vi "Write Project Item.vi"(10 "Project Item":refnum<vi>, 11 "Target Store in":refnum<class "Target Store.lvclass">) -> (3 "Target Store out":refnum<class "Target Store.lvclass">)   [LabVIEW 2020, in "Add Actor.lvlib" / "Target Store.lvclass"]
uses:
  Target Store.lvclass
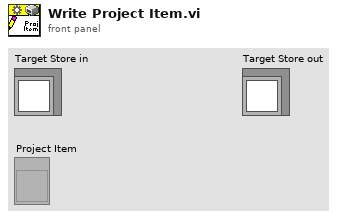
[diagram p1: front panel]
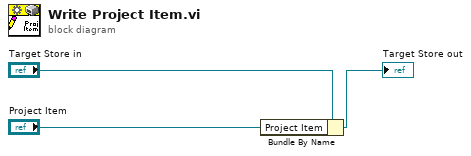
[diagram p0: block diagram]
diagram:
  n1 = Bundle By Name(cluster="Target Store in", "Project Item"="Project Item") -> (→"Target Store out":refnum<class "Target Store.lvclass">)
